vi "Write Test.vi"(6 "Test":string, 11 "Executioner in":refnum<class "Executioner.lvclass">) -> (3 "Executioner out":refnum<class "Executioner.lvclass">)   [LabVIEW 2019, in "Test Executive.lvlib" / "Executioner.lvclass"]
uses:
  <vilib>/gpm_packages/@cs/test-executive/Source/Test Executive/Executioner/Executioner.lvclass
  <vilib>/gpm_packages/@cs/test-executive/Source/Test Executive/Executioner/Executioner.lvclass/Executioner.ctl
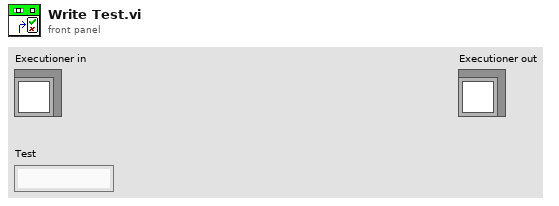
[diagram p1: front panel]
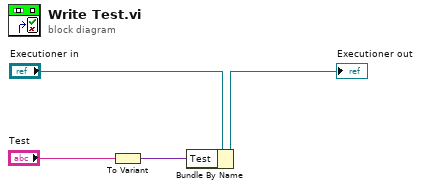
[diagram p0: block diagram]
diagram:
  n1 = To Variant(anything="Test") -> (Variant=w1:variant)
  n2 = Bundle By Name(cluster="Executioner in", "Test"=w1) -> (→"Executioner out":refnum<class "Executioner.lvclass">)
